vi "Test Motors.vi"() -> ()   [LabVIEW 2011]
uses:
  <vilib>/robotics/Starter Kit/1.0/9631 Host Interface/NI_Robotics_Starter Kit Host_9631_1.0.lvclass
  <vilib>/robotics/Utilities/RPM to Radians per Second (Scalar).vi
  <vilib>/robotics/Utilities/Radians per Second to RPM (Scalar).vi
  <vilib>/robotics/Utilities/NI_Robotics Utilities.lvlib
  <vilib>/robotics/Starter Kit/Host Interface/NI_Robotics_Starter Kit Host.lvclass
panel:
  in  "Left":dbl(slide) min=-100.0 max=100.0 step=4.0 scale=-70.0..70.0
  in  "Right":dbl(slide) min=-100.0 max=100.0 step=4.0 scale=-70.0..70.0
  out "Wheel Velocities (rpm)":cluster{"Left":dbl, dbl, "Right":dbl, dbl}(graph)
  in  "stop":bool
  # "Caution:  Moving the sliders will drive the robot.  Please ensure that it can safely move before continuing.\n\nTurn the MOTORS switch on, then move the sliders to control the forward wheel velocities in RPM."
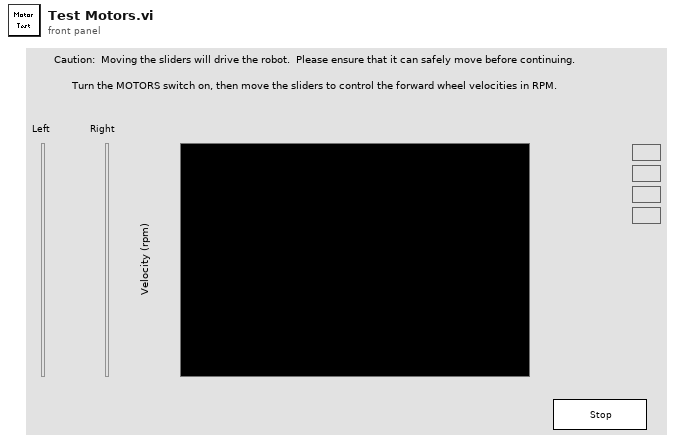
[diagram p1: front panel]
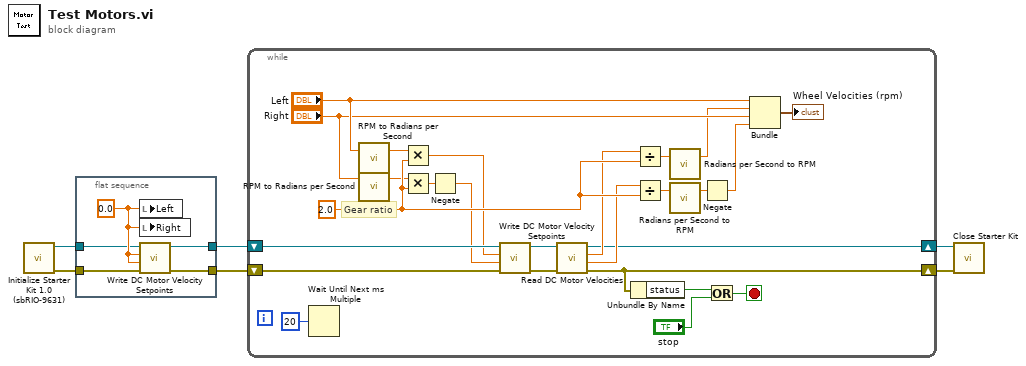
[diagram p0: block diagram]
diagram:
  n1 = call <vilib>:"Initialize Starter Kit 1.0 (sbRIO-9631).vi"() -> ("error out"=w2:errorcluster, "FPGA starter kit host 1.0 out"=w1:refnum<class "NI_Robotics_Starter Kit Host_9631_1.0.lvclass">)  [unwired: 10 in]
  n2 = flat-sequence {
    tunnel: w1 -> [w10]
    tunnel: w2 -> [w7]
    tunnel: [w9] -> w6
    tunnel: [w8] -> w5
    frame #0 {
      w11 = 0.0 ("left ccw motor velocity (rad/s)")
      n3 = local write "Left"(w11) -> ()
      n4 = local write "Right"(w11) -> ()
      n5 = call <vilib>:"Write DC Motor Velocity Setpoints.vi"("error in (no error)"=w7, "right motor ccw velocity (rad/s)"=w11, "left motor ccw velocity (rad/s)"=w11, "starter kit host in"=w10) -> ("error out"=w8:errorcluster, "starter kit host out"=w9:refnum<class "NI_Robotics_Starter Kit Host_9631_1.0.lvclass">)  [unwired: 6 in]
    }
  }
  n6 = while {
    shift-right: [w12] -> w3
    shift-left: w5 -> [w18]
    shift-right: [w13] -> w4
    shift-left: w6 -> [w21]
    stop <- w36 stop-if-true
    w31 = 2.0 ("y")
    # "Gear ratio"
    n7 = Wait Until Next ms Multiple(millisecond multiple=u32 20) -> ()  [unwired: 1 out]
    n8 = call-poly <vilib>:"RPM to Radians per Second.vi"("rpm"="Left") -> ("radians per second"=w29:dbl)  [unwired: 2 in]
    n9 = call-poly <vilib>:"RPM to Radians per Second.vi"("rpm"="Right") -> ("radians per second"=w27:dbl)  [unwired: 2 in]
    n10 = Multiply(x=w29, y=w31) -> (x*y=w20:dbl)
    n11 = Multiply(x=w27, y=w31) -> (x*y=w33:dbl)
    n12 = Negate(x=w33) -> (-x=w19:dbl)
    n13 = call <vilib>:"Write DC Motor Velocity Setpoints.vi"("error in (no error)"=w18, "right motor ccw velocity (rad/s)"=w19, "left motor ccw velocity (rad/s)"=w20, "starter kit host in"=w21) -> ("error out"=w14:errorcluster, "starter kit host out"=w15:refnum<class "NI_Robotics_Starter Kit Host_9631_1.0.lvclass">)  [unwired: 6 in]
    n14 = call <vilib>:"Read DC Motor Velocities.vi"("error in (no error)"=w14, "starter kit host in"=w15) -> ("error out"=w12:errorcluster, "right motor ccw velocity (rad/s)"=w16:dbl, "left motor ccw velocity (rad/s)"=w17:dbl, "starter kit host out"=w13:refnum<class "NI_Robotics_Starter Kit Host_9631_1.0.lvclass">)  [unwired: 6 in]
    n15 = Unbundle By Name(w12) -> ("status"=w37:bool)
    n16 = Divide(x=w17, y=w31) -> (x/y=w26:dbl)
    n17 = Divide(x=w16, y=w31) -> (x/y=w25:dbl)
    n18 = call-poly <vilib>:"Radians per Second to RPM.vi"("radians per second"=w26) -> ("rpm"=w24:dbl)  [unwired: 2 in]
    n19 = call-poly <vilib>:"Radians per Second to RPM.vi"("radians per second"=w25) -> ("rpm"=w32:dbl)  [unwired: 2 in]
    n20 = Negate(x=w32) -> (-x=w23:dbl)
    n21 = Or(x=w37, y="stop") -> (x .or. y?=w36:bool)
    n22 = Bundle("Left"="Left", "rpm"=w24, "Right"="Right", w23) -> (→"Wheel Velocities (rpm)":cluster{"Left":dbl, "rpm":dbl, "Right":dbl, dbl})  [unwired: 1 in]
  }
  n23 = call-dynamic "Close Starter Kit.vi"("error in (no error)"=w3, "starter kit host in"=w4) -> ()  [unwired: 9 in, 1 out]
